vi "InsertDB.vi"(7 "Boolean":bool=TRUE, 9 "String":string, 10 "Entity":string) -> (1 "error out":errorcluster)   [LabVIEW 2012]
uses:
  <vilib>/addons/database/Connection.llb/DB Tools Open Connec (Path).vi
  <vilib>/Utility/file.llb/Read From Spreadsheet File (string).vi
  <vilib>/Utility/file.llb/Read From Spreadsheet File (I64).vi
  <vilib>/addons/database/NI_Database_API.lvlib
panel:
  out "output cluster":T1
  out "before substring 9":string
  in  "input cluster":T1
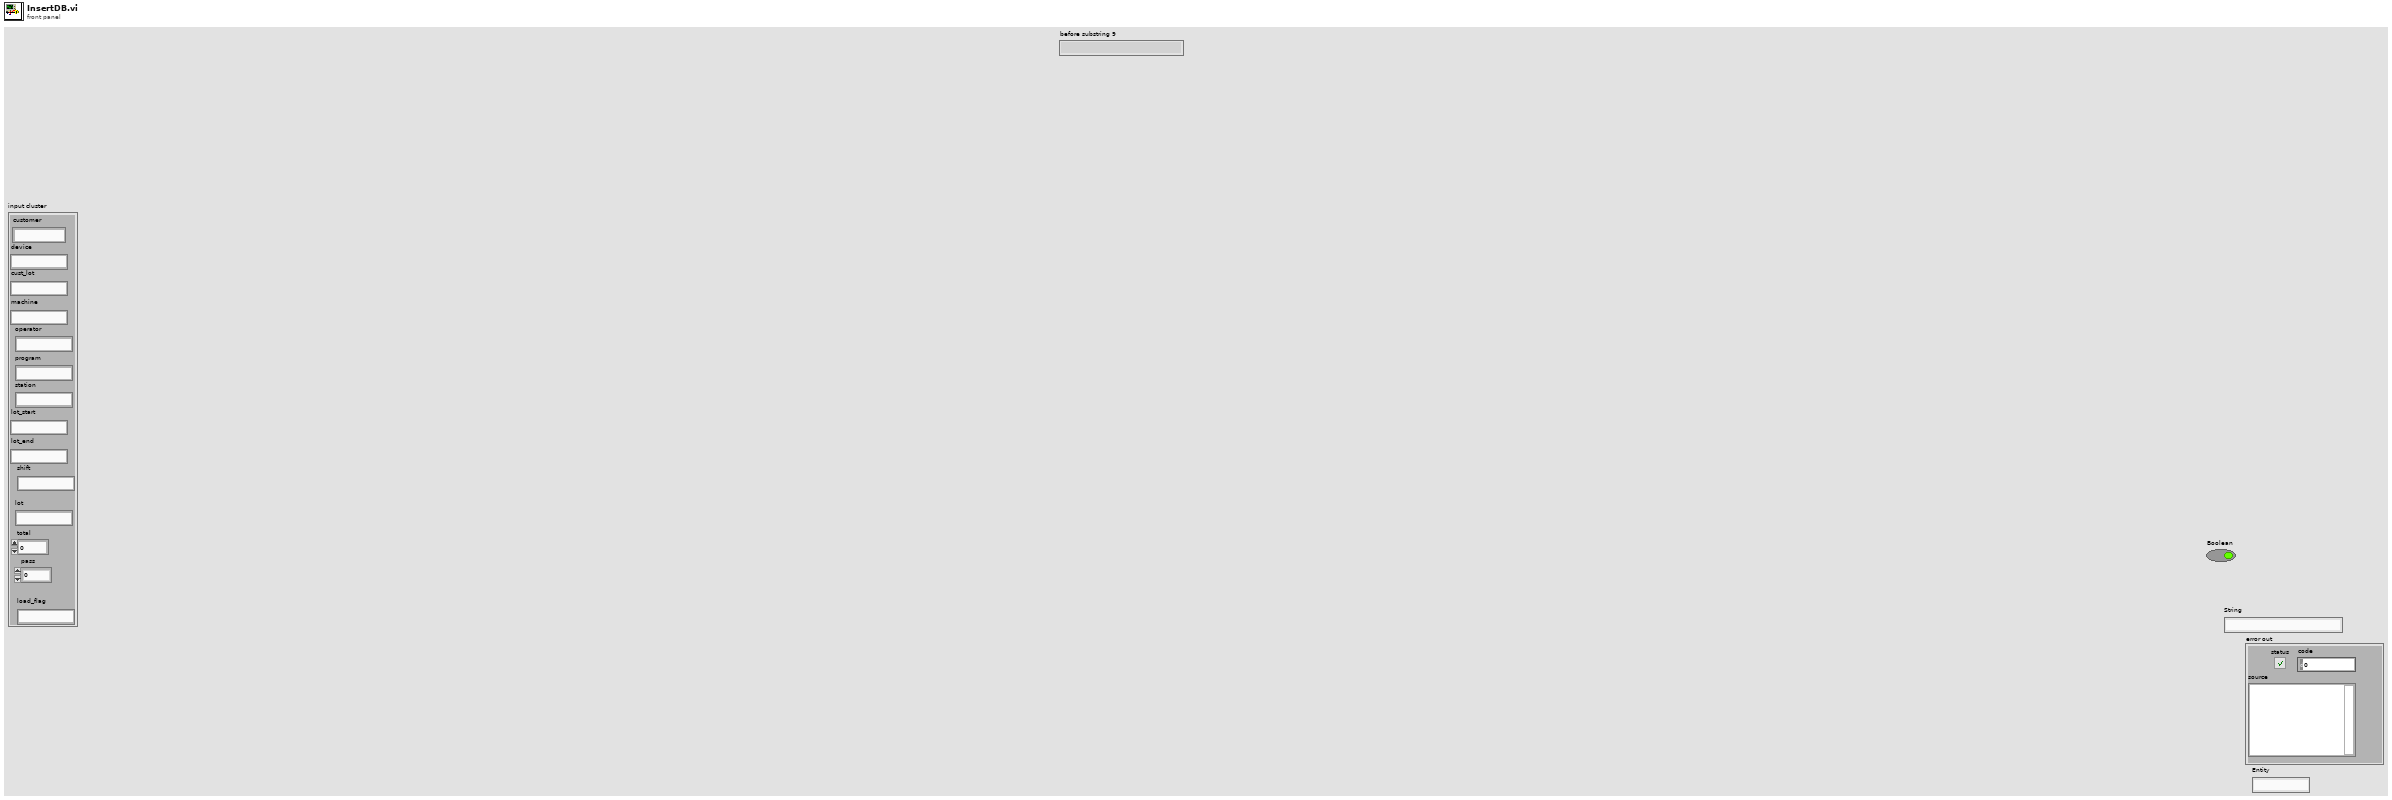
[diagram p1: front panel]
types:
  T1 = cluster{"customer":string, "device":string, "cust_lot":string, "machine":string, "operator":string, "program":string, "station":string, "lot_start":string, "lot_end":string, "shift":string, "lot":string, "total":dbl, "pass":dbl, "load_flag":string}
  T2 = typedef "NI_Database_API.lvlib/Conn ObjectReference.ctl" = refnum<k1>
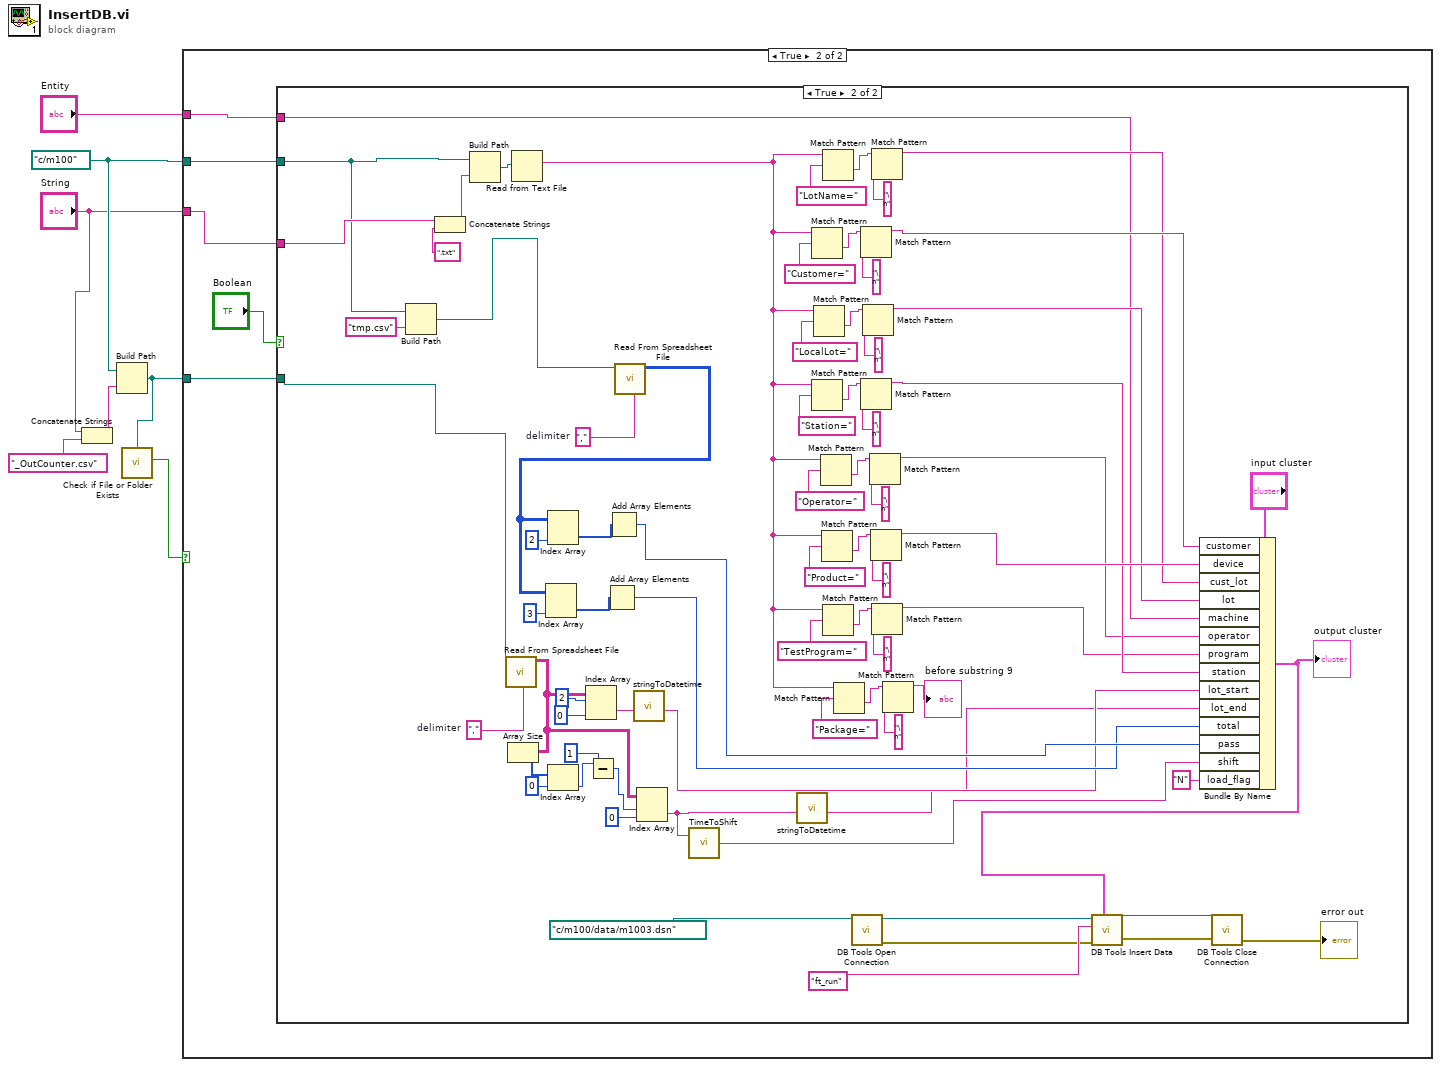
[diagram p0: block diagram]
diagram:
  w4 = path "c:/m100" ("base path")
  n1 = Concatenate Strings("String", "_OutCounter.csv" ("string")) -> (w5:string)
  n2 = Build Path(base path=w4, name or relative path=w5) -> (appended path=w3:path)
  n3 = call <vilib>:"Check if File or Folder Exists.vi"("path"=w3) -> ("file or folder exists?"=w2:bool)  [unwired: 8 in, 2 out]
  n4 = case shown="True" w2 {
    tunnel: "Entity" -> [_ w11]
    tunnel: "String" -> [_ w10]
    tunnel: w4 -> [_ w9]
    tunnel: w3 -> [_ w8]
    frame False {
    }
    frame True {
      n5 = case shown="True" "Boolean" {
        tunnel: w9 -> [_ w28]
        tunnel: w10 -> [_ w42]
        tunnel: w11 -> [_ w23]
        tunnel: w8 -> [_ w13]
        frame False {
        }
        frame True {
          w41 = ","  # delimiter
          w58 = ","  # delimiter
          n6 = Build Path(base path=w28, name or relative path="tmp.csv") -> (appended path=w26:path)
          n7 = Concatenate Strings(w42, ".txt" ("string")) -> (w87:string)
          n8 = Build Path(base path=w28, name or relative path=w87) -> (appended path=w84:path)
          n9 = call-poly <vilib>:"Read From Spreadsheet File.vi"("delimiter (\\t)"=w41, "file path (dialog if empty)"=w13) -> ("all rows"=w30:string[][])  [unwired: 5 in, 4 out]
          n10 = Array Size(array=w30) -> (size(s)=w36:i32[])
          n11 = Read from Text File(file (use dialog)=w84) -> (text=w59:string)  [unwired: 3 in, 3 out]
          n12 = Index Array(array=w36, index=0) -> (element=w33:i32)
          n13 = Index Array(array=w30, index (row)=2 ("disabled index (row)"), index (col)=0 ("disabled index (col)")) -> (element=w38:string)
          n14 = Subtract(x=w33, y=1) -> (x-y=w31:i32)
          n15 = call-poly <vilib>:"Read From Spreadsheet File.vi"("delimiter (\\t)"=w58, "file path (dialog if empty)"=w26) -> ("all rows"=w53:i64[][])  [unwired: 5 in, 4 out]
          n16 = Index Array(array=w53, index (col)=3 ("disabled index (col)")) -> (element=w54:i64[])  [unwired: 1 in]
          n17 = Index Array "Index Array"(array=w53, index (col)=2 ("disabled index (col)")) -> (element=w56:i64[])  [unwired: 1 in]
          n18 = Add Array Elements(numeric array=w54) -> (sum=w43:i64)
          n19 = Add Array Elements(numeric array=w56) -> (sum=w44:i64)
          n20 = call "stringToDatetime.vi"("input string"=w38) -> ("date/time string"=w37:string)  [unwired: 10 in]
          n21 = Index Array(array=w30, index (row)=w31, index (col)=0 ("disabled index (col)")) -> (element=w21:string)
          n22 = call "TimeToShift.vi"("input string"=w21) -> ("s? t:f"=w22:string)  [unwired: 1 in]
          n23 = call "stringToDatetime.vi"("input string"=w21) -> ("date/time string"=w29:string)  [unwired: 10 in]
          n24 = Match Pattern(string=w59, regular expression="Customer=") -> (after substring=w80:string)  [unwired: 1 in, 3 out]
          n25 = Match Pattern(string=w59, regular expression="Station=") -> (after substring=w74:string)  [unwired: 1 in, 3 out]
          n26 = Match Pattern(string=w59, regular expression="LocalLot=") -> (after substring=w77:string)  [unwired: 1 in, 3 out]
          n27 = Match Pattern(string=w59, regular expression="Operator=") -> (after substring=w71:string)  [unwired: 1 in, 3 out]
          n28 = Match Pattern(string=w59, regular expression="Product=") -> (after substring=w68:string)  [unwired: 1 in, 3 out]
          n29 = Match Pattern(string=w59, regular expression="LotName=") -> (after substring=w83:string)  [unwired: 1 in, 3 out]
          n30 = Match Pattern(string=w59, regular expression="TestProgram=") -> (after substring=w65:string)  [unwired: 1 in, 3 out]
          n31 = Match Pattern(string=w59, regular expression="Package=") -> (after substring=w62:string)  [unwired: 1 in, 3 out]
          n32 = call-poly <vilib>:"DB Tools Open Connection.vi"("connection information"=path "c:/m100/data/m1003.dsn") -> ("error out"=w15:errorcluster, "connection reference"=w16:T2)  [unwired: 7 in]
          n33 = Match Pattern(string=w80, regular expression="\n") -> (before substring=w51:string)  [unwired: 1 in, 3 out]
          n34 = Match Pattern(string=w74, regular expression="\n") -> (before substring=w47:string)  [unwired: 1 in, 3 out]
          n35 = Match Pattern(string=w77, regular expression="\n") -> (before substring=w48:string)  [unwired: 1 in, 3 out]
          n36 = Match Pattern(string=w71, regular expression="\n") -> (before substring=w46:string)  [unwired: 1 in, 3 out]
          n37 = Match Pattern(string=w68, regular expression="\n") -> (before substring=w50:string)  [unwired: 1 in, 3 out]
          n38 = Match Pattern(string=w83, regular expression="\n") -> (before substring=w49:string)  [unwired: 1 in, 3 out]
          n39 = Match Pattern(string=w65, regular expression="\n") -> (before substring=w45:string)  [unwired: 1 in, 3 out]
          n40 = Match Pattern(string=w62, regular expression="\n") -> (before substring=→"before substring 9":string)  [unwired: 1 in, 3 out]
          n41 = Bundle By Name(cluster="input cluster", "customer"=w51, "device"=w50, "cust_lot"=w49, "lot"=w48, "machine"=w23, "operator"=w46, "program"=w45, "station"=w47, "lot_start"=w37, "lot_end"=w29, "total"=w43, "pass"=w44, "shift"=w22, "load_flag"="N") -> (w19:T1)
          "output cluster" <- w19
          n42 = call <vilib>:"DB Tools Insert Data.vi"("data"=w19, "error in (no error)"=w15, "table"="ft_run", "connection reference"=w16) -> ("error out"=w17:errorcluster, "connection reference out"=w18:T2)  [unwired: 6 in]
          n43 = call <vilib>:"DB Tools Close Connection.vi"("error in (no error)"=w17, "connection reference"=w18) -> ("error out"=→"error out":errorcluster)  [unwired: 5 in]
        }
      }
    }
  }
